vi "Root Actor Class Is Loaded.vi"(8 "error in (no error)":errorcluster, 11 "TargetItem in":refnum<vi>) -> (0 "error out":errorcluster, 2 "is Actor.lvclass loaded already?":bool, 3 "TargetItem out":refnum<vi>)   [LabVIEW 2020, in "Message Maker.lvlib"]
uses:
  Message Maker.lvlib
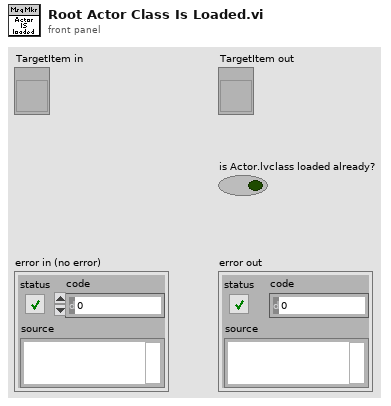
[diagram p1: front panel]
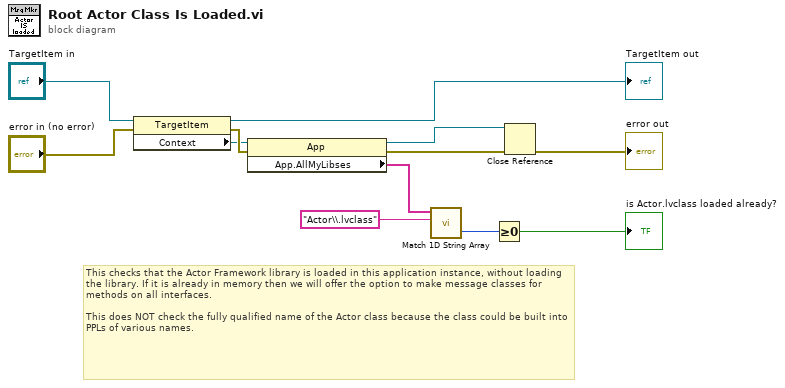
[diagram p0: block diagram]
diagram:
  # "This checks that the Actor Framework library is loaded in this application instance, without loading the library. If it is already in memory then we will offer the option to make message classes for methods on all interfaces.\n\nThis does NOT check the fully qualified name of the Actor class because the class could be built into PPLs of various names."
  n1 = property class="TargetItem"(reference="TargetItem in", error in="error in (no error)") -> (reference out=→"TargetItem out":refnum<vi>, error out=w10:errorcluster, "Context"=w6:refnum<vi>)
  n2 = property class="App"(reference=w6, error in=w10) -> (reference out=w8:refnum<vi>, error out=w9:errorcluster, "App.AllMyLibses"=w4:string[])
  n3 = call <vilib>:"Match 1D String Array.vi"("Pattern"="Actor\\.lvclass" ("element"), "Strings"=w4) -> ("index of element"=w2:i32)  [unwired: 2 in, 1 out]
  n4 = Greater Or Equal To 0?(x=w2) -> (x >= 0?=→"is Actor.lvclass loaded already?":bool)
  n5 = Close Reference(reference=w8, error in (no error)=w9) -> (error out=→"error out":errorcluster)
